vi "RSZVB Get Frequency LO Conversion Factor.vi"(8 "error in (no error)":errorcluster {"code" format="%.0x"}, 9 "Stage (1)":i32=1, 10 "Channel (1)":i32=1, 11 "VISA resource name":refnum<visa-resource-name>) -> (0 "error out":errorcluster {"code" format="%.0x"}, 1 "Denominator":i32, 2 "Numerator":i32, 3 "VISA resource name out":refnum<visa-resource-name>)   [LabVIEW 2011]
doc: "This VI queries the frequency conversion factors for the LO 1 or L0 2 signal.\n\nRemote-control command(s):\n[SENSe<Ch>:]FREQuency:CONVersion:MIXer:LOMultiplier<Stg>?"
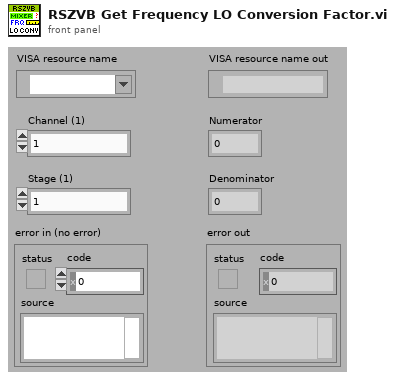
[diagram p1: front panel]
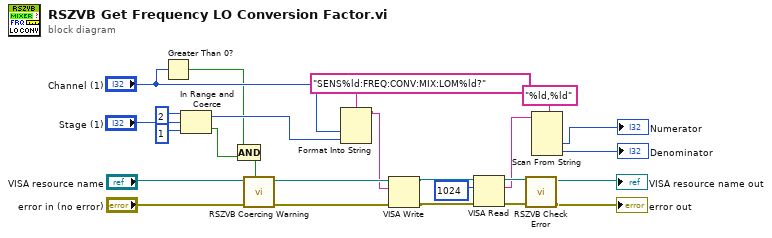
[diagram p0: block diagram]
diagram:
  n1 = Greater Than 0?(x="Channel (1)") -> (x > 0?=w7:bool)
  n2 = In Range and Coerce(upper limit=2, x="Stage (1)", lower limit=1) -> (coerced(x)=w9:i32, In Range?=w8:bool)
  n3 = Compound Arithmetic op=AND(w7, w8) -> (w23:bool)
  n4 = call "RSZVB Coercing Warning.vi"("In Range?"=w23, "error in (no error)"="error in (no error)", "VISA session"="VISA resource name") -> ("error out"=w24:errorcluster, "dup VISA session"=w25:refnum<visa-resource-name>)  [unwired: 7 in]
  n5 = Format Into String(format string="SENS%ld:FREQ:CONV:MIX:LOM%ld?", "Channel (1)", w9) -> (resulting string=w21:string)  [unwired: 2 in, 1 out]
  n6 = VISA Write(VISA resource name=w25, write buffer=w21, error in (no error)=w24) -> (VISA resource name out=w17:refnum<visa-resource-name>, error out=w16:errorcluster)  [unwired: 1 out]
  n7 = VISA Read(VISA resource name=w17, byte count=u32 1024 ("byte count (0)"), error in (no error)=w16) -> (VISA resource name out=w15:refnum<visa-resource-name>, read buffer=w12:string, error out=w14:errorcluster)  [unwired: 1 out]
  n8 = call "RSZVB Check Error.vi"("error in (no error)"=w14, "VISA session"=w15) -> ("error out"=→"error out":errorcluster, "dup VISA session"=→"VISA resource name out":refnum<visa-resource-name>)  [unwired: 8 in]
  n9 = Scan From String(format string="%ld,%ld", input string=w12) -> (output 1=→"Numerator":i32, output 2=→"Denominator":i32)  [unwired: 4 in, 3 out]
